vi "_PC_Pub_PeakFinding.vi"(8 "error in (no error)":errorcluster, 10 "XY Cluster in":cluster{"X":dbl[], "Y":dbl[]}) -> (0 "error out":errorcluster, 1 "# found":i32, 2 "Annotation":T1(array[cluster]))   [LabVIEW 2018]
uses:
  <vilib>/Analysis/baseanly.llb/Unimode.vi
  <vilib>/Analysis/NI_AAL_SigProc.lvlib
  <vilib>/Analysis/NI_AALBase.lvlib
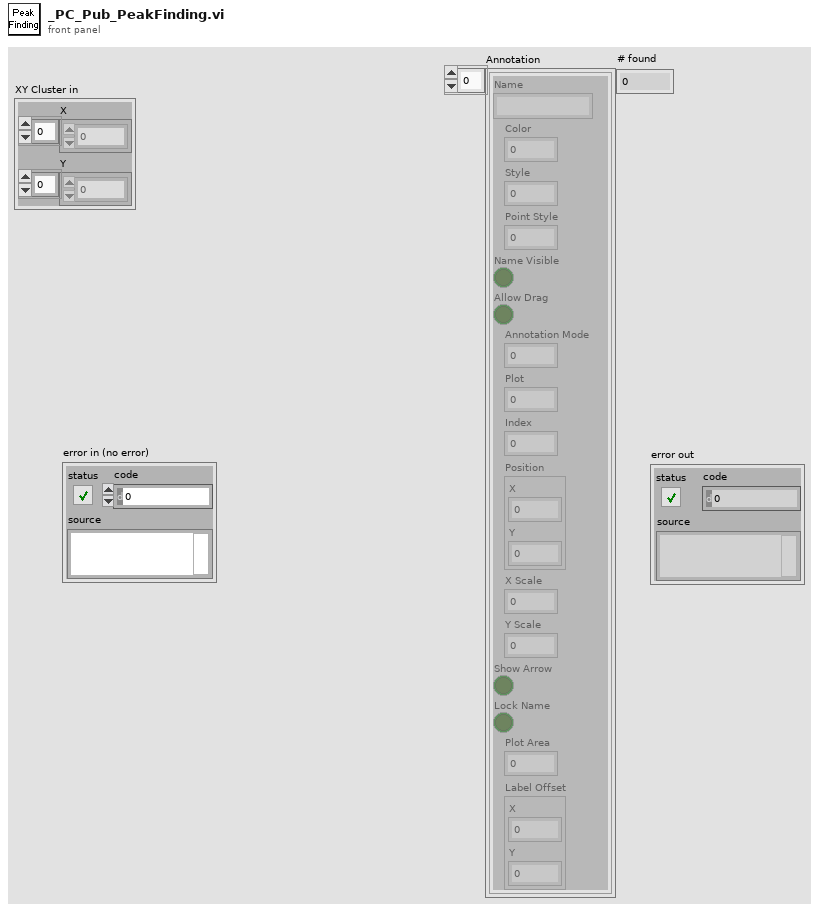
[diagram p1: front panel]
types:
  T1 = cluster{"Name":string, "Color":u32, "Style":u8, "Point Style":u8, "Name Visible":bool, "Allow Drag":bool, "Annotation Mode":u32, "Plot":i32, "Index":i32, "Position":cluster{"X":dbl, "Y":dbl}, "X Scale":u32, "Y Scale":u32, "Show Arrow":bool, "Lock Name":bool, "Plot Area":i32, "Label Offset":cluster{"X":dbl, "Y":dbl}}[]
  T2 = cluster{"Name":string, "Color":u32, "Style":u8, "Point Style":u8, "Name Visible":bool, "Allow Drag":bool, "Annotation Mode":u32, "Plot":i32, "Index":i32, "Position":cluster{"X":dbl, "Y":dbl}, "X Scale":u32, "Y Scale":u32, "Show Arrow":bool, "Lock Name":bool, "Plot Area":i32, "Label Offset":cluster{"X":dbl, "Y":dbl}}
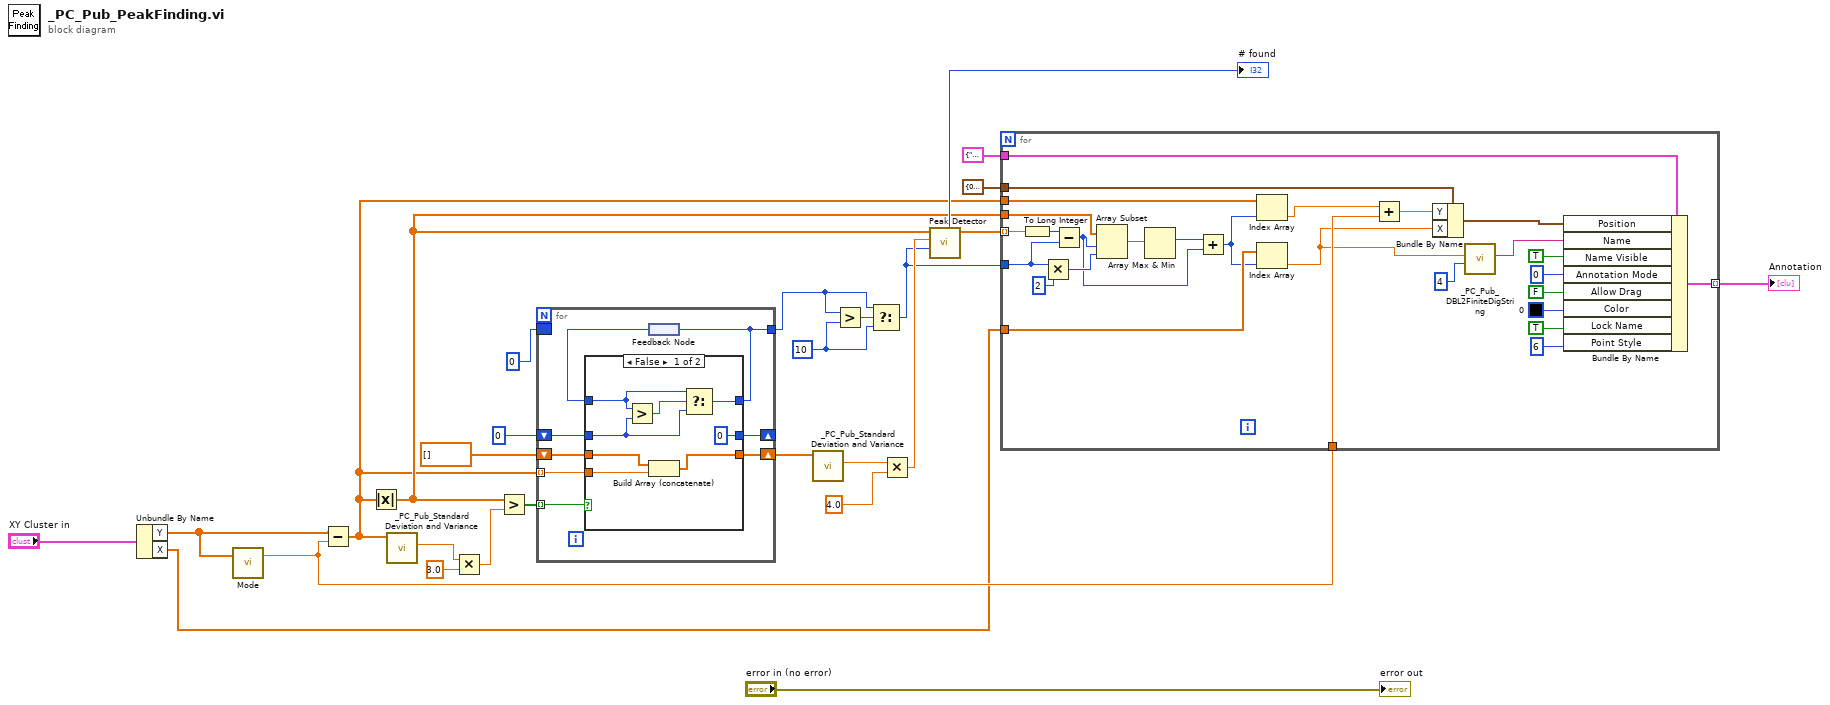
[diagram p0: block diagram]
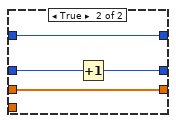
[diagram p2: hidden frame]
diagram:
  w7 = 10 ("y")
  n1 = Unbundle By Name("XY Cluster in") -> ("Y"=w15:dbl[], "X"=w13:dbl[])
  n2 = call-poly <vilib>:"Mode.vi"("X"=w15) -> ("mode"=w14:dbl)  [unwired: 1 in, 1 out]
  n3 = Subtract(x=w15, y=w14) -> (x-y=w4:dbl[])
  n4 = Absolute Value(x=w4) -> (abs(x)=w10:dbl[])
  n5 = call "_PC_Pub_Standard Deviation and Variance.vi"("X"=w4) -> ("standard deviation"=w3:dbl)  [unwired: 8 in, 2 out]
  n6 = Multiply(x=w3, y=3.0) -> (x*y=w25:dbl)
  n7 = Greater?(x=w10, y=w25) -> (0:w24:bool[])
  n8 = for {
    tunnel: w24 -> [w33] mode=indexing
    shift-right: [w34] -> _
    shift-left: 0 -> [w35]
    shift-right: [w31] -> w2
    shift-left: dbl[] [] -> [w30]
    tunnel: w4 -> [w32] mode=indexing
    border: 0 -> [_]
    tunnel: [w28] -> w8
    n9 = feedback #1() -> (w29:i32)
    n10 = case shown="False" w33 {
      tunnel: w35 -> [w41 w47]
      tunnel: [0 w46] -> w34
      tunnel: w32 -> [w36 _]
      tunnel: [w37 w44] -> w31
      tunnel: w30 -> [w38 w44]
      tunnel: [w40 w45] -> w28
      tunnel: w29 -> [w39 w45]
      frame False {
        n11 = Greater?(x=w39, y=w41) -> (0:w42:bool)
        n12 = Build Array (concatenate)(w38, w36) -> (w37:dbl[])
        n13 = Select(t=w39, s=w42, f=w41) -> (s? t:f=w40:i32)
      }
      frame True {
        n14 = Increment(x=w47) -> (x+1=w46:i32)
      }
    }
    n15 = feedback-in #1(w28) -> ()
  }
  n16 = call "_PC_Pub_Standard Deviation and Variance.vi"("X"=w2) -> ("standard deviation"=w1:dbl)  [unwired: 8 in, 2 out]
  n17 = Greater?(x=w8, y=w7) -> (0:w9:bool)
  n18 = Select(t=w8, s=w9, f=w7) -> (s? t:f=w6:i32)
  n19 = Multiply(x=w1, y=4.0) -> (x*y=w11:dbl)
  n20 = call <vilib>:"Peak Detector.vi"("width"=w6, "threshold"=w11, "X"=w10) -> ("Locations"=w20:dbl[], "# found"=→"# found":i32)  [unwired: 4 in, 3 out]
  n21 = for {
    tunnel: w20 -> [w63] mode=indexing
    tunnel: w10 -> [w60]
    tunnel: cluster{"X":dbl, "Y":dbl} {"X"=0.0, "Y"=0.0} ("Position") -> [w75]
    tunnel: T2 {"Name"="", "Color"=0, "Style"=0, "Point Style"=0, "Name Visible"=FALSE, "Allow Drag"=FALSE, "Annotation Mode"=0, "Plot"=0, "Index"=0, "Position"={"X"=0.0, "Y"=0.0}, "X Scale"=0, "Y Scale"=0, "Show Arrow"=FALSE, "Lock Name"=FALSE, "Plot Area"=0, "Label Offset"={"X"=0.0, "Y"=0.0}} -> [w74]
    tunnel: [w68] -> w5 mode=indexing
    tunnel: w14 -> [w64]
    tunnel: w13 -> [w56]
    tunnel: w6 -> [w57]
    tunnel: w4 -> [w55]
    n22 = To Long Integer(number=w63) -> (32bit integer=w52:i32)
    n23 = Multiply(x=w57, y=2) -> (x*y=w61:i32)
    n24 = Subtract(x=w52, y=w57) -> (x-y=w53:i32)
    n25 = Array Subset(array=w60, index=w53, length=w61) -> (w59:dbl[])
    n26 = Array Max & Min(array=w59) -> (max index (indices)=w58:i32)  [unwired: 3 out]
    n27 = Add(x=w58, y=w53) -> (x+y=w54:i32)
    n28 = Index Array(array=w55, index=w54) -> (element=w48:dbl)
    n29 = Index Array(array=w56, index=w54) -> (element=w51:dbl)
    n30 = Add(x=w48, y=w64) -> (x+y=w65:dbl)
    n31 = Bundle By Name(cluster=w75, "Y"=w65, "X"=w51) -> (w73:cluster{"X":dbl, "Y":dbl})
    n32 = call "_PC_Pub_DBL2FiniteDigString.vi"("Digit"=4, "DBL in"=w51) -> ("String out"=w50:string)  [unwired: 9 in]
    n33 = Bundle By Name(cluster=w74, "Position"=w73, "Name"=w50, "Name Visible"=TRUE, "Annotation Mode"=u32 0, "Allow Drag"=FALSE, "Color"=u32 0, "Lock Name"=TRUE, "Point Style"=u8 6) -> (w68:T2)
  }
  "Annotation" <- w5
  "error out" <- "error in (no error)"
